vi "Rename.vi"(6 "Options":T1={"Atomic"=TRUE, "Native"=TRUE, "Overwrite"=TRUE}, 8 "Error In":errorcluster, 9 "Remote Destination Path":string, 10 "Remote Source Path":string, 11 "SFTP In":refnum<class "SFTP.lvclass">) -> (0 "Error Out":errorcluster, 3 "SFTP Out":refnum<class "SFTP.lvclass">)   [LabVIEW 2021, in "Field_RnD_Services_LIBSSH2_Toolkit.lvlib" / "SFTP.lvclass"]
doc: "Changes the name of a filesystem entry on the remote SFTP server. This is also an alias for moving a filesystem entry on the remote SFTP server."
uses:
  SFTP.lvclass
  Type Definitions/Rename Options.ctl
  SFTP.lvclass/SFTP.ctl
  Field_RnD_Services_LIBSSH2_Toolkit.lvlib
  Session/Session.lvclass
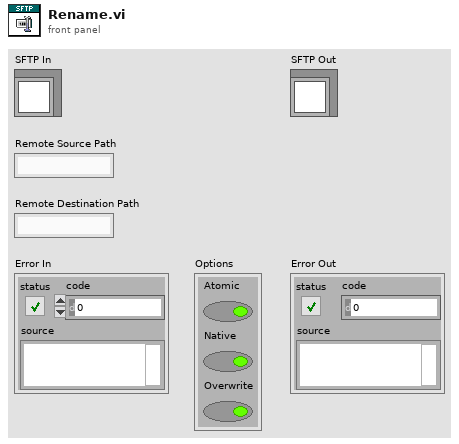
[diagram p1: front panel]
types:
  T1 = typedef "Field_RnD_Services_LIBSSH2_Toolkit.lvlib/SFTP.lvclass/Rename Options.ctl" = cluster{"Atomic":bool, "Native":bool, "Overwrite":bool}
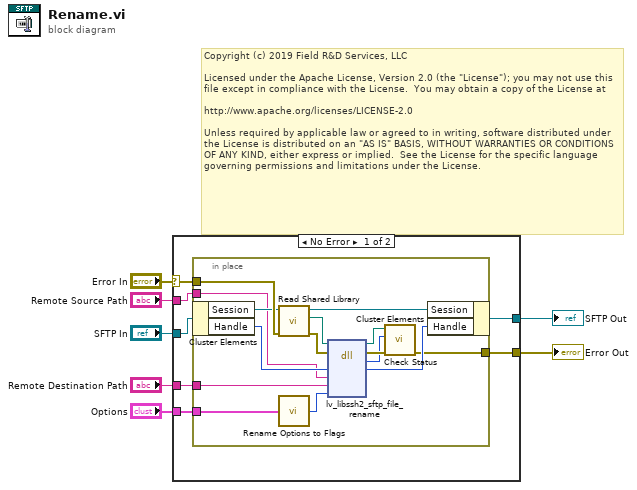
[diagram p0: block diagram]
diagram:
  # "Copyright (c) 2019 Field R&D Services, LLC\n\nLicensed under the Apache License, Version 2.0 (the \"License\"); you may not use this file except in compliance with the License.  You may obtain a copy of the License at\n\nhttp://www.apache.org/licenses/LICENSE-2.0\n\nUnless required by applicable law or agreed to in writing, software distributed under the License is distributed on an \"AS IS\" BASIS, WITHOUT WARRANTIES OR CONDITIONS OF ANY KIND, either express or implied.  See the License for the specific language governing permissions and limitations under the License."
  n1 = case shown="No Error" "Error In" {
    selector: "Error In" -> [w14 w31]
    tunnel: [w13 w31] -> w6
    tunnel: "SFTP In" -> [w12 w30]
    tunnel: [w11 w30] -> w4
    tunnel: "Remote Source Path" -> [w10 _]
    tunnel: "Remote Destination Path" -> [w9 _]
    tunnel: "Options" -> [w8 _]
    frame No Error {
      n2 = in-place {
        in-place-border: w14 -> [w24]
        in-place-border: [w25] -> w13
        in-place-border: w10 -> [w18]
        in-place-border: w9 -> [w17]
        in-place-border: w8 -> [w16]
        n3 = in-place-cluster #1(w12) -> ("Session"=w23:refnum<class "Session.lvclass">, "Handle"=w19:u64)
        n4 = call "Read Shared Library.vi"("Error In"=w24, "Session In"=w23) -> ("Erorr Out"=w21:errorcluster, "libssh2lv Shared Library"=w20:path, "Session Out"=w22:refnum<class "Session.lvclass">)  [unwired: 7 in]
        n5 = call "Rename Options to Flags.vi"("Options"=w16) -> ("Flags"=w15:i32)
        n6 = dll-call lib="libssh2lv.*" fn="lv_libssh2_sftp_file_rename"(path in=w20, error in=w21, "handle"=w19, "source_path"=w18, "destination_path"=w17, "options"=w15) -> (path out=w27:path, error out=w28:errorcluster, "status"=w26:i32, "handle"=w29:u64)  [unwired: 4 in]
        n7 = call "Check Status.vi"("Error In"=w28, "Status"=w26, "libssh2lv Shared Library In"=w27) -> ("Error Out"=w25:errorcluster)  [unwired: 7 in, 1 out]
        n8 = in-place-cluster #1("Session"=w22, "Handle"=w29) -> (w11:refnum<class "SFTP.lvclass">)
      }
    }
    frame Error {
    }
  }
  "Error Out" <- w6
  "SFTP Out" <- w4
